vi "Progress Window.vi"(8 "error in (no error)":errorcluster, 11 "queue":refnum<queue>) -> (0 "error out":errorcluster)   [LabVIEW 2017, in "DSF System Explorer.lvlib"]
uses:
  DSF System Explorer.lvlib
  progress window data.ctl
panel:
  out "message":string
  out "progress":dbl(slide) scale=0.0..1.0
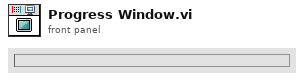
[diagram p1: front panel]
types:
  T1 = typedef "DSF System Explorer.lvlib/progress window data.ctl" = cluster{"stop":bool, "message":string, "progress":dbl}
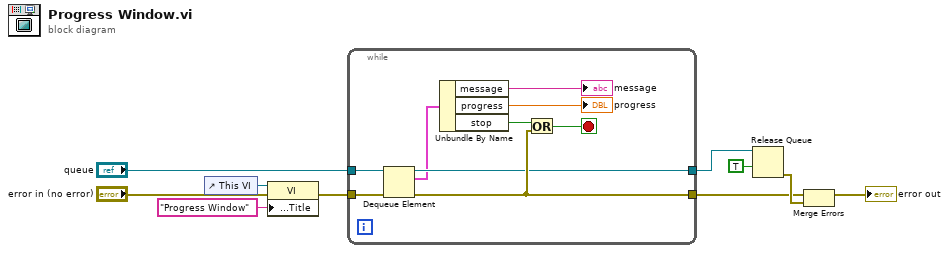
[diagram p0: block diagram]
diagram:
  n1 = control-ref of="This VI"() -> (w4:refnum<vi>)
  n2 = property class="VI"(reference=w4, error in="error in (no error)", "Front Panel.Title"="Progress Window" ("Front Panel Window:Title")) -> (error out=w2:errorcluster)  [unwired: 1 out]
  n3 = while {
    tunnel: "queue" -> [w19]
    tunnel: w2 -> [w18]
    tunnel: [w17] -> w6
    tunnel: [w12] -> w9
    stop <- w13 stop-if-true
    n4 = Dequeue Element(queue=w19, error in (no error)=w18) -> (queue out=w12:refnum<queue>, element=w11:T1, error out=w17:errorcluster)  [unwired: 1 in, 1 out]
    n5 = Unbundle By Name(w11) -> ("message"=→"message":string, "progress"=→"progress":dbl, "stop"=w16:bool)
    n6 = Or(x=w16, y=w17) -> (x .or. y?=w13:bool)
  }
  n7 = Release Queue(queue=w9, force destroy? (F)=TRUE) -> (error out=w7:errorcluster)  [unwired: 1 in, 2 out]
  n8 = Merge Errors(w6, w7) -> (→"error out":errorcluster)
